vi "RM-absolute-motion.vi"(8 "error in (no error)":errorcluster, 10 "position to go":dbl, 11 "MB_Master_Serial输入":refnum<class "MB_Master_Serial.lvclass">) -> (0 "error out":errorcluster, 3 "MB_Master_Serial输出":refnum<class "MB_Master_Serial.lvclass">)   [LabVIEW 2014]
uses:
  <vilib>/Plasmionique/MB Master/MB_Master_Serial/MB_Master_Serial.lvclass
  <vilib>/Plasmionique/MB Master/MB Master.lvlib
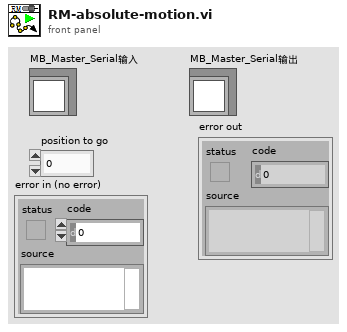
[diagram p1: front panel]
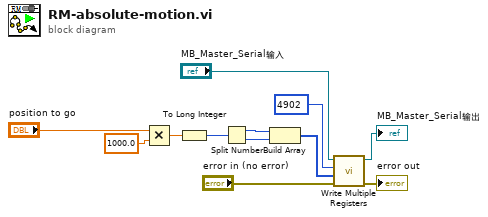
[diagram p0: block diagram]
diagram:
  n1 = Multiply(x="position to go", y=1000.0) -> (x*y=w6:dbl)
  n2 = To Long Integer(number=w6) -> (32bit integer=w7:i32)
  n3 = Split Number(x=w7) -> (hi(x)=w8:u16, lo(x)=w9:u16)
  n4 = Build Array(w8, w9) -> (w4:u16[])
  n5 = call <vilib>:"Write Multiple Registers.vi"("error in (no error)"="error in (no error)", "values"=w4, "starting address"=u16 4902, "MB session in"="MB_Master_Serial输入") -> ("error out"=→"error out":errorcluster, "MB session out"=→"MB_Master_Serial输出":refnum<class "MB_Master_Serial.lvclass">)  [unwired: 6 in]
